vi "Create From Template.vi"() -> ()   [LabVIEW 2021]
uses:
  _Create From Template/_Create From Template.lvlib
  _Create From Template/Script Strategy/Second Library Script Strategy/Second Library Script Strategy.lvclass
panel:
  in  "Template":string(combo)
  in  "Name":string
  in  "Create":bool
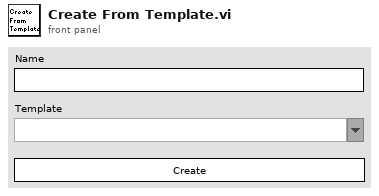
[diagram p1: front panel]
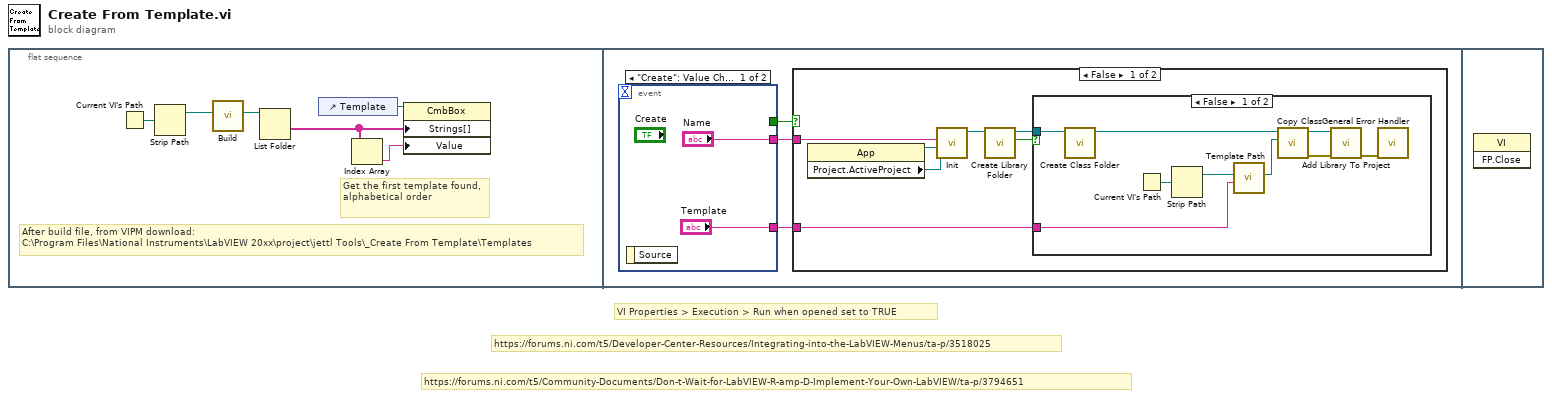
[diagram p0: block diagram]
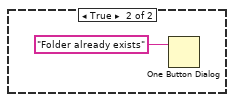
[diagram p2: hidden frame]
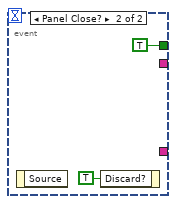
[diagram p4: hidden frame]
diagram:
  # "https://forums.ni.com/t5/Community-Documents/Don-t-Wait-for-LabVIEW-R-amp-D-Implement-Your-Own-LabVIEW/ta-p/3794651"
  # "https://forums.ni.com/t5/Developer-Center-Resources/Integrating-into-the-LabVIEW-Menus/ta-p/3518025"
  # "VI Properties > Execution > Run when opened set to TRUE"
  n1 = flat-sequence {
    frame #0 {
      # "After build file, from VIPM download:\nC:\\Program Files\\National Instruments\\LabVIEW 20xx\\project\\jettl Tools\\_Create From Template\\Templates"
      # "Get the first template found, alphabetical order"
      n2 = Current VI's Path() -> (path=w4:path)
      n3 = Strip Path(path=w4) -> (stripped path=w3:path)  [unwired: 1 out]
      n4 = call "Build.vi"("Base Path"=w3) -> ("Templates Path"=w2:path)  [unwired: 10 in]
      n5 = List Folder(path=w2) -> (folder names=w1:string[])  [unwired: 3 in, 3 out]
      n6 = control-ref of="Template"() -> (w5:refnum<vi>)
      n7 = Index Array(array=w1) -> (element=w6:string)  [unwired: 1 in]
      n8 = property class="CmbBox"(reference=w5, "Strings[]"=w1, "Value"=w6) -> ()  [unwired: 1 in, 2 out]
    }
    frame #1 {
      n9 = event shown="[0] \"Create\": Value Change" {
        selector: _ -> [_ _]
        dyn-events: _ -> [_ _]
        timeout: _ -> [_ _]
        tunnel: ["Name" _] -> w9
        tunnel: [_ TRUE] -> w8
        tunnel: ["Template" _] -> w7
        event "Create": Value Change {
          n10 = event-data() -> ()  [unwired: 1 in, 1 out]
        }
        event Panel Close? {
          n11 = event-data() -> ()  [unwired: 1 in, 1 out]
          n12 = event-data("Discard?"=TRUE) -> ()  [unwired: 1 in, 1 out]
        }
      }
      n13 = case shown="False" w8 {
        tunnel: w9 -> [w16 _]
        tunnel: w7 -> [w10 _]
        frame False {
          n14 = property class="App"() -> (reference out=w15:refnum<vi>, "Project.ActiveProject"=w14:refnum<vi>)  [unwired: 2 in, 1 out]
          n15 = call-dynamic "Init.vi"("Project:Active Project"=w14, "Application Instance"=w15, "Name"=w16) -> ("Second Library Script Strategy out"=w13:refnum<class "Second Library Script Strategy.lvclass">)  [unwired: 8 in]
          n16 = call-dynamic "Create Library Folder.vi"("Second Library Script Strategy in"=w13) -> ("Library Folder Already Exists?"=w11:bool, "Second Library Script Strategy out"=w12:refnum<class "Second Library Script Strategy.lvclass">)  [unwired: 9 in]
          n17 = case shown="False" w11 {
            tunnel: w12 -> [w20 _]
            tunnel: w10 -> [w18 _]
            frame False {
              n18 = call-dynamic "Create Class Folder.vi"("Second Library Script Strategy in"=w20) -> ("Second Library Script Strategy out"=w19:refnum<class "Second Library Script Strategy.lvclass">)  [unwired: 10 in]
              n19 = Current VI's Path() -> (path=w25:path)
              n20 = Strip Path(path=w25) -> (stripped path=w17:path)  [unwired: 1 out]
              n21 = call "Template Path.vi"("Template Name"=w18, "Base Path"=w17) -> ("Template Path"=w24:path)  [unwired: 9 in]
              n22 = call-dynamic "Copy Class.vi"("Template Path"=w24, "Second Library Script Strategy in"=w19) -> ("error out"=w22:errorcluster, "Second Library Script Strategy out"=w21:refnum<class "Second Library Script Strategy.lvclass">)  [unwired: 8 in]
              n23 = call-dynamic "Add Library To Project.vi"("error in"=w22, "Second Library Script Strategy in"=w21) -> ("error out"=w23:errorcluster)  [unwired: 9 in]
              n24 = call <vilib>:"General Error Handler.vi"("error in (no error)"=w23) -> ()  [unwired: 10 in, 5 out]
            }
            frame True {
              n25 = One Button Dialog(message="Folder already exists") -> ()  [unwired: 1 in, 1 out]
            }
          }
        }
        frame True {
        }
      }
    }
    frame #2 {
      n26 = invoke class="VI" method="FP.Close"() -> ()  [unwired: 3 in, 3 out]
    }
  }
